vi "PH_SSAC.check Background.vi"(0 "i ref in":refnum<vi>, 5 "error in":errorcluster) -> (14 "i ref out":refnum<vi>, 15 "BG ok?":bool, 16 "dt [fs]":dbl, 17 "BG.Background Calibration Data.Signal":dbl[](array[numeric]), 18 "Calibration Factor [fs/pixel]":dbl, 19 "error out":errorcluster)   [LabVIEW 2014, in "PH_SSAC.lvlib"]
uses:
  PH_SSAC.lvlib
  PH_Common/PH_Common.lvlib
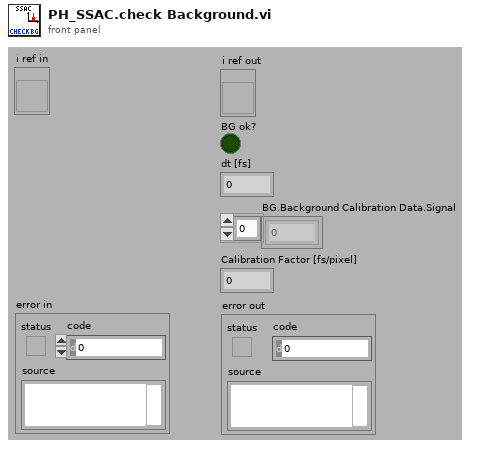
[diagram p1: front panel]
types:
  T1 = typedef "PH_SSAC.lvlib/PH_SSAC.i attribute.ctl" = cluster{"GUI Refs":cluster{"Delete":refnum<vi>, "Global On":refnum<vi>, "Cam Source":refnum<vi>, "Frame Main Signal":refnum<vi>, "Frame Background":refnum<vi>, "dt (Gauss smooth)":refnum<vi>, "Calibration Factor":refnum<vi>, "Background acquire":refnum<vi>, "Threshold":refnum<vi>, "Time evolution of mean pulse duration":refnum<vi>, "Mean Pulse Duration":refnum<vi>, "Main signal":refnum<vi>, "Current Pulse Duration":refnum<vi>, "Processed":refnum<vi>, "Saturation":refnum<vi>, "# for Average":refnum<vi>, "Position":refnum<vi>, "BG Status":refnum<vi>, "Save BG data":refnum<vi>, "Read BG Data":refnum<vi>, "Background Calibration Data":refnum<vi>}, "Images":cluster{"OP Image":T2, "GUI Image":T2, "PSDB Image":T2}, "Global On?":bool, "Frame Main":cluster{"x":u32, "dx":u32, "y":u32, "dy":u32}, "Frame Background":cluster{"x":u32, "dx":u32, "y":u32, "dy":u32}, "dt [fs]":dbl, "Calibration Factor [fs/pixel]":dbl, "Threshold":dbl, "Time evolution of mean pulse duration [fs]":dbl[], "Main Signal":cluster{"Time for Main":dbl[], "Signal":dbl[]}, "Processed":bool, "Current Pulse Duration [fs]":dbl, "# for Average":i32, "Position":i32, "Pulse Durations [fs]":dbl[], "BG":cluster{"Acquire?":bool, "Background Calibration Data":T3, "Save Data":bool}}
  T2 = typedef "IMAQ Image.ctl" = refnum<image>
  T3 = typedef "PH_SSAC.lvlib/PH_SSAC.Background Data.ctl" = cluster{"Date":string, "Time":string, "Frame Main":cluster{"x":u32, "dx":u32, "y":u32, "dy":u32}, "dt [fs]":dbl, "Calibration Factor [fs/pixel]":dbl, "Signal":dbl[], "Frame Background":cluster{"x":u32, "dx":u32, "y":u32, "dy":u32}}
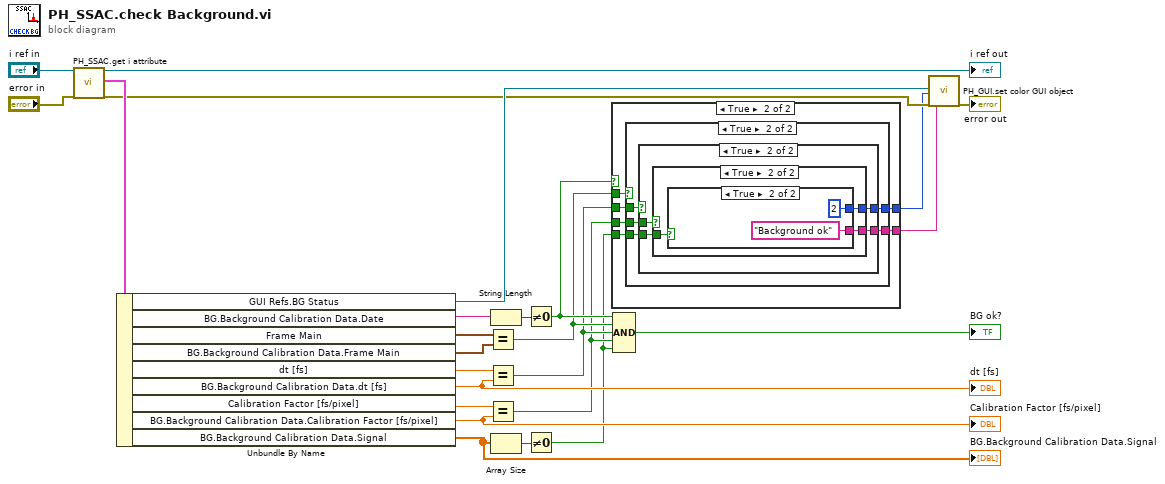
[diagram p0: block diagram]
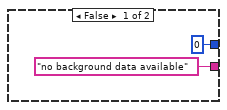
[diagram p2: hidden frame]
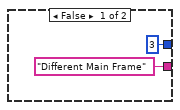
[diagram p3: hidden frame]
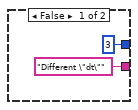
[diagram p4: hidden frame]
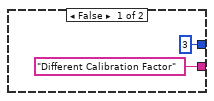
[diagram p5: hidden frame]
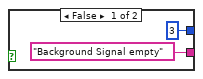
[diagram p6: hidden frame]
diagram:
  n1 = call "PH_SSAC.get i attribute.vi"("i ref in"="i ref in", "error in (no error)"="error in") -> ("i ref out"=→"i ref out":refnum<vi>, "i attribute"=w22:T1, "error out"=w14:errorcluster)  [unwired: 15 in]
  n2 = Unbundle By Name(w22) -> ("GUI Refs.BG Status"=w15:refnum<vi>, "BG.Background Calibration Data.Date"=w8:string, "Frame Main"=w21:cluster{"x":u32, "dx":u32, "y":u32, "dy":u32}, "BG.Background Calibration Data.Frame Main"=w20:cluster{"x":u32, "dx":u32, "y":u32, "dy":u32}, "dt [fs]"=w19:dbl, "BG.Background Calibration Data.dt [fs]"=w18:dbl, "Calibration Factor [fs/pixel]"=w17:dbl, "BG.Background Calibration Data.Calibration Factor [fs/pixel]"=w16:dbl, "BG.Background Calibration Data.Signal"=w12:dbl[])
  "dt [fs]" <- w18
  "Calibration Factor [fs/pixel]" <- w16
  "BG.Background Calibration Data.Signal" <- w12
  n3 = Equal?(x=w21, y=w20) -> (x = y?=w6:bool)
  n4 = Equal?(x=w19, y=w18) -> (x = y?=w3:bool)
  n5 = Equal?(x=w17, y=w16) -> (x = y?=w2:bool)
  n6 = String Length(string=w8) -> (length=w10:i32)
  n7 = Array Size(array=w12) -> (size(s)=w11:i32)
  n8 = Not Equal To 0?(x=w10) -> (x != 0?=w7:bool)
  n9 = Not Equal To 0?(x=w11) -> (x != 0?=w1:bool)
  n10 = case shown="True" w7 {
    tunnel: w6 -> [_ w33]
    tunnel: [0 ("State") w31] -> w5
    tunnel: ["no background data available" w32] -> w4
    tunnel: w3 -> [_ w30]
    tunnel: w2 -> [_ w29]
    tunnel: w1 -> [_ w28]
    frame False {
    }
    frame True {
      n11 = case shown="True" w33 {
        tunnel: ["Different Main Frame" w39] -> w32
        tunnel: [3 ("State") w38] -> w31
        tunnel: w30 -> [_ w40]
        tunnel: w29 -> [_ w37]
        tunnel: w28 -> [_ w36]
        frame False {
        }
        frame True {
          n12 = case shown="True" w40 {
            tunnel: ["Different \"dt\"" w44] -> w39
            tunnel: [3 ("State") w45] -> w38
            tunnel: w37 -> [_ w46]
            tunnel: w36 -> [_ w43]
            frame False {
            }
            frame True {
              n13 = case shown="True" w46 {
                tunnel: [3 ("State") w51] -> w45
                tunnel: ["Different Calibration Factor" w50] -> w44
                tunnel: w43 -> [_ w49]
                frame False {
                }
                frame True {
                  n14 = case shown="True" w49 {
                    tunnel: [3 ("State") 2 ("State")] -> w51
                    tunnel: ["Background Signal empty" "Background ok"] -> w50
                    frame False {
                    }
                    frame True {
                    }
                  }
                }
              }
            }
          }
        }
      }
    }
  }
  n15 = Compound Arithmetic op=AND(w7, w6, w3, w2, w1) -> (→"BG ok?":bool)
  n16 = call "PH_GUI.set color GUI object.vi"("GUI object Ref"=w15, "State"=w5, "error in (no error)"=w14, "Tip Strip (N/A)"=w4) -> ("error out"=→"error out":errorcluster)  [unwired: 15 in]
